vi "Config File Test.vi"() -> ()   [LabVIEW 2016]
uses:
  Classes/Config_Read/Frame_Data.ctl
  Classes/Config_Read/OperationMode.ctl
  Classes/Config_Read/BurstLength.ctl
  Classes/Config_Read/RW_Option.ctl
  Classes/Config_Read/Config_Read_BML.lvclass
panel:
  out "FRM_Data_Array":T1[](array[typedef]) {"Data" format="%x"; "Start_Addr" format="%x"}
  out "error out":errorcluster
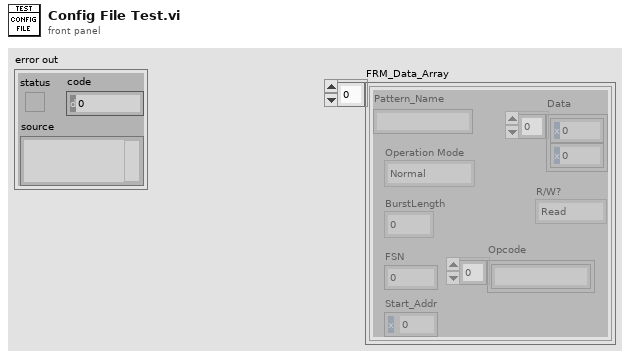
[diagram p1: front panel]
types:
  T1 = typedef "Config_Read_BML.lvclass/Frame_Data.ctl" = cluster{"Pattern_Name":string, "Operation Mode":T2, "BurstLength":T3, "FSN":u8, "Start_Addr":u16, "Data":u8[], "R/W?":T4, "Opcode":string[]}
  T2 = typedef "Config_Read_BML.lvclass/OperationMode.ctl" = enum8{"Normal", "ImmeEffect", "InitSlaveID", "LoadData"}
  T3 = typedef "Config_Read_BML.lvclass/BurstLength.ctl" = enum8{"0", "2", "3", "4", "5", "8", "16", "32"}
  T4 = typedef "Config_Read_BML.lvclass/RW_Option.ctl" = enum16{"Read", "Write", "R/W"}
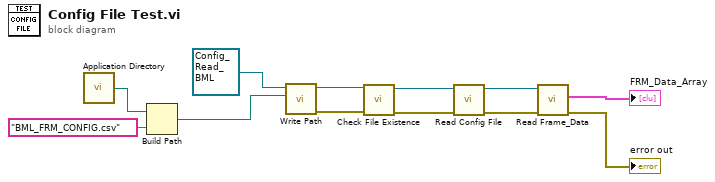
[diagram p0: block diagram]
diagram:
  n1 = call <vilib>:"Application Directory.vi"() -> ("Application Directory"=w3:path)
  n2 = Build Path(base path=w3, name or relative path="BML_FRM_CONFIG.csv") -> (appended path=w1:path)
  n3 = call-dynamic "Write Path.vi"("Path"=w1, "Config_Read in"=refnum<class "Config_Read_BML.lvclass"> refnum ("Config_Read.lvclass")) -> ("error out"=w10:errorcluster, "Config_Read out"=w11:refnum<class "Config_Read_BML.lvclass">)  [unwired: 8 in]
  n4 = call-dynamic "Check File Existence.vi"("error in (no error)"=w10, "Config_Read in"=w11) -> ("error out"=w8:errorcluster, "Config_Read out"=w9:refnum<class "Config_Read_BML.lvclass">)  [unwired: 8 in]
  n5 = call-dynamic "Read Config File.vi"("error in (no error)"=w8, "Config_Read in"=w9) -> ("error out"=w6:errorcluster, "Config_Read out"=w7:refnum<class "Config_Read_BML.lvclass">)  [unwired: 8 in]
  n6 = call-dynamic "Read Frame_Data.vi"("error in (no error)"=w6, "Config_Read in"=w7) -> ("error out"=→"error out":errorcluster, "FRM_Data_Array"=→"FRM_Data_Array":T1[])  [unwired: 7 in, 1 out]
